vi "13-2.vi"() -> ()   [LabVIEW 2019, in "13.lvlib"]
uses:
  13.lvlib
panel:
  out "sum":i16
  out "Array 3":i32[](array[numeric])
  out "Array 2":string[](array[string])
  out "Array":bool[][](array[boolean])
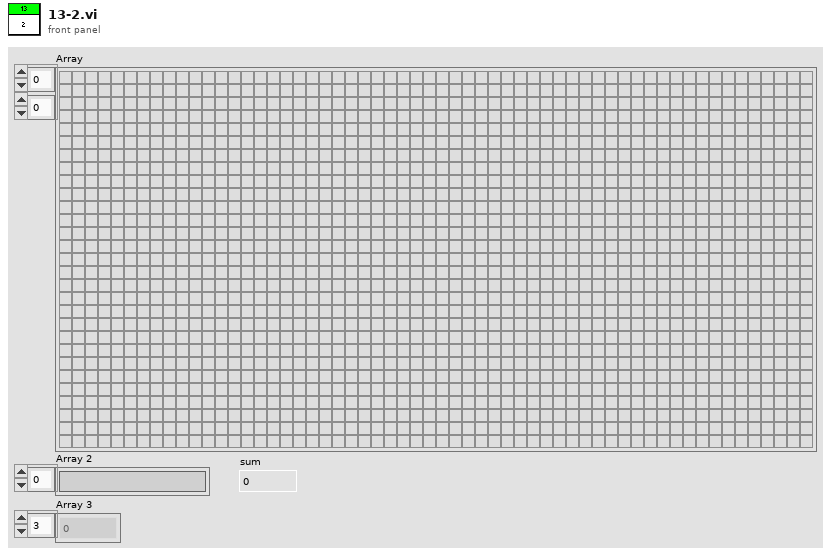
[diagram p1: front panel]
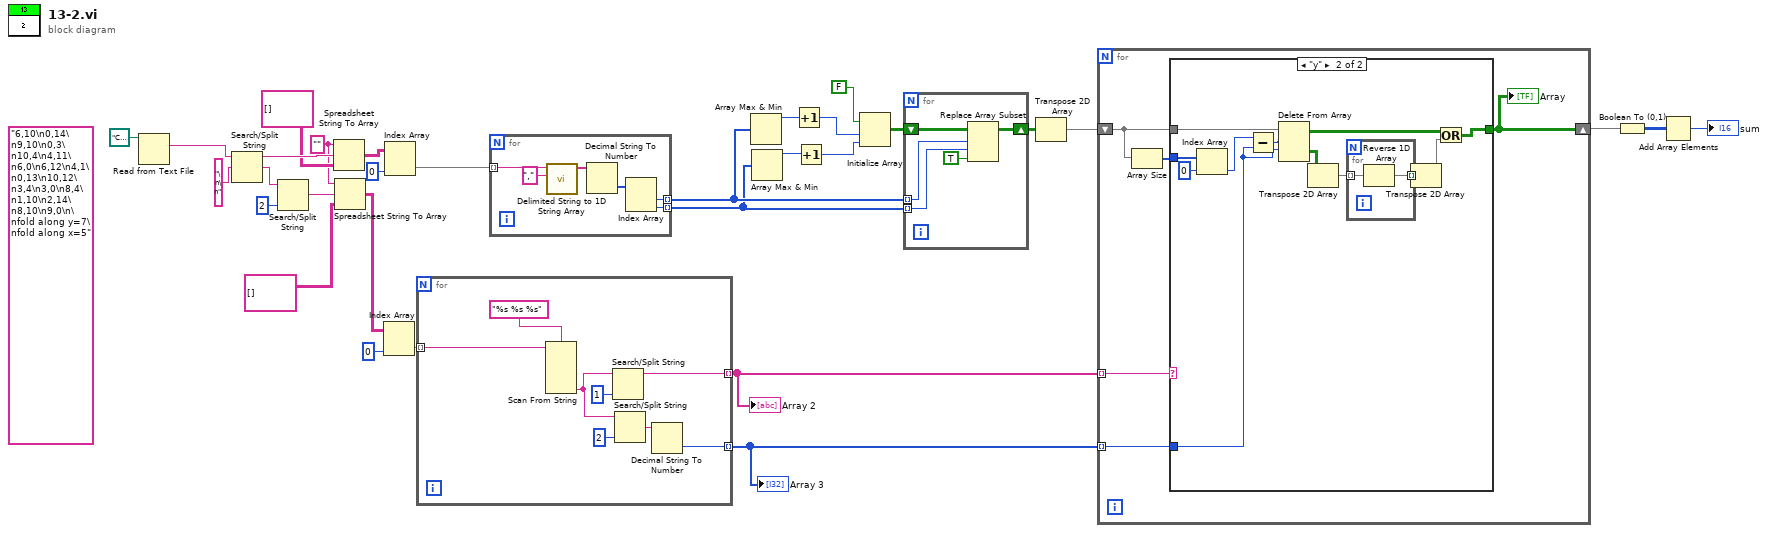
[diagram p0: block diagram]
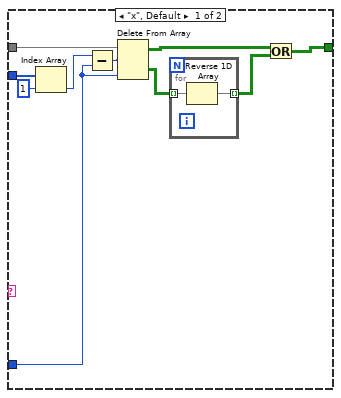
[diagram p2: hidden frame]
diagram:
  w26 = "" ("format string")
  (unwired) "6,10\n0,14\n9,10\n0,3\n10,4\n4,11\n6,0\n6,12\n4,1\n0,13\n10,12\n3,4\n3,0\n8,4\n1,10\n2,14\n8,10\n9,0\n\nfold along y=7\nfold along x=5"
  n1 = Read from Text File(file (use dialog)=path "C:/Users/craig.walker/Documents/GitHub/lv2019-Advent-of-Code-2021/13/input.txt") -> (text=w5:string)  [unwired: 3 in, 3 out]
  n2 = Search/Split String(string=w5, search string/char (-)="\n\n") -> (substring before match=w30:string, match + rest of string=w29:string)  [unwired: 1 in, 1 out]
  n3 = Search/Split String(string=w29, offset (0)=2) -> (match + rest of string=w10:string)  [unwired: 1 in, 2 out]
  n4 = Spreadsheet String To Array(format string=w26, spreadsheet string=w30, array type (2D Dbl)=string[][] []) -> (array=w25:string[][])  [unwired: 1 in]
  n5 = Spreadsheet String To Array(format string=w26, spreadsheet string=w10, array type (2D Dbl)=string[][] [] ("match + rest of string")) -> (array=w23:string[][])  [unwired: 1 in]
  n6 = Index Array(array=w23, index (col)=0 ("disabled index (col)")) -> (element=w11:string[])  [unwired: 1 in]
  n7 = Index Array(array=w25, index (col)=0 ("disabled index (col)")) -> (element=w21:string[])  [unwired: 1 in]
  n8 = for {
    tunnel: w11 -> [w39] mode=indexing
    tunnel: [w36] -> w8 mode=indexing
    tunnel: [w32] -> w7 mode=indexing
    n9 = Scan From String(format string="%s %s %s", input string=w39) -> (output 3=w35:string)  [unwired: 7 in, 3 out]
    n10 = Search/Split String(string=w35, offset (0)=1) -> (substring before match=w36:string)  [unwired: 1 in, 2 out]
    n11 = Search/Split String(string=w35, offset (0)=2) -> (match + rest of string=w33:string)  [unwired: 1 in, 2 out]
    n12 = Decimal String To Number(string=w33) -> (number=w32:i32)  [unwired: 2 in, 1 out]
  }
  "Array 2" <- w8
  "Array 3" <- w7
  n13 = for {
    tunnel: w21 -> [w45] mode=indexing
    tunnel: [w41] -> w14 mode=indexing
    tunnel: [w40] -> w13 mode=indexing
    n14 = call <vilib>:"Delimited String to 1D String Array.vi"("delimiter"=",", "delimited string"=w45) -> ("string array"=w43:string[])  [unwired: 9 in]
    n15 = Decimal String To Number(string=w43) -> (number=w42:i32[])  [unwired: 2 in, 1 out]
    n16 = Index Array(array=w42) -> (element #1=w41:i32, element #2=w40:i32)  [unwired: 2 in]
  }
  n17 = Array Max & Min(array=w14) -> (max value=w20:i32)  [unwired: 3 out]
  n18 = Array Max & Min(array=w13) -> (max value=w19:i32)  [unwired: 3 out]
  n19 = Increment(x=w20) -> (x+1=w17:i32)
  n20 = Increment(x=w19) -> (x+1=w16:i32)
  n21 = Initialize Array(FALSE, w17, w16) -> (w15:bool[][])
  n22 = for {
    shift-right: [w49] -> w12
    shift-left: w15 -> [w50]
    tunnel: w14 -> [w47] mode=indexing
    tunnel: w13 -> [w48] mode=indexing
    n23 = Replace Array Subset(array=w50, new element=TRUE ("new element/subarray"), index (row)=w47, index (col)=w48) -> (w49:bool[][])
  }
  n24 = Transpose 2D Array(2D array=w12) -> (transposed array=w6:bool[][])
  n25 = for {
    tunnel: w8 -> [w55] mode=indexing
    tunnel: w7 -> [w54] mode=indexing
    shift-right: [w51] -> w3
    shift-left: w6 -> [w53]
    n26 = Array Size(array=w53) -> (size(s)=w52:i32[])
    n27 = case shown="\"y\"" w55 {
      tunnel: w54 -> [w61 w71]
      tunnel: w53 -> [w65 w79]
      tunnel: w52 -> [w64 w78]
      tunnel: [w57 w72] -> w51
      frame "x", Default {
        n28 = Index Array(array=w64, index=1) -> (element=w62:i32)
        n29 = Subtract(x=w62, y=w61) -> (x-y=w60:i32)
        n30 = Delete From Array(array=w65, length=w60, index (col)=w61) -> (deleted portion=w58:bool[][], array with subset deleted=w59:bool[][])  [unwired: 1 in]
        n31 = for {
          tunnel: w58 -> [w67] mode=indexing
          tunnel: [w66] -> w56 mode=indexing
          n32 = Reverse 1D Array(array=w67) -> (reversed array=w66:bool[])
        }
        n33 = Or(x=w59, y=w56) -> (x .or. y?=w57:bool[][])
      }
      frame "y" {
        n34 = Index Array(array=w78, index=0) -> (element=w76:i32)
        n35 = Subtract(x=w76, y=w71) -> (x-y=w75:i32)
        n36 = Delete From Array(array=w79, length=w75, index (row)=w71) -> (deleted portion=w73:bool[][], array with subset deleted=w74:bool[][])  [unwired: 1 in]
        n37 = Transpose 2D Array(2D array=w73) -> (transposed array=w69:bool[][])
        n38 = for {
          tunnel: w69 -> [w81] mode=indexing
          tunnel: [w80] -> w70 mode=indexing
          n39 = Reverse 1D Array(array=w81) -> (reversed array=w80:bool[])
        }
        n40 = Transpose 2D Array(2D array=w70) -> (transposed array=w68:bool[][])
        n41 = Or(x=w74, y=w68) -> (x .or. y?=w72:bool[][])
      }
    }
    "Array" <- w51
  }
  n42 = Boolean To (0,1)(Boolean=w3) -> (0, 1=w2:i16[][])
  n43 = Add Array Elements(numeric array=w2) -> (sum=→"sum":i16)
